vi "McPherson Control.vi"() -> ()   [LabVIEW 2020]
uses:
  Globals and TypeDefs/Type Definitions.llb/McPherson Status.ctt
  Globals and TypeDefs/Type Definitions.llb/Wavelength Unit.ctt
  Globals and TypeDefs/Type Definitions.llb/McPherson Grating Density.ctl
  Globals and TypeDefs/Error Categories.ctt
  Globals and TypeDefs/gSpectrometer.vi
  Instance          17 25Saved   McPherson Control .vi
panel:
  in  "Case Constant\n(See Context Help)":bool
  in  "Spectrometer Pos":T2
  in  "Done":bool
  in  "Tab Control":enum32{"Regular Display", "For Experts ONLY"}(tab)
  out "Speed":dbl=10.0 caption="nm/s" format="%#_3g"
  out "Lambda Chart":dbl(graph)
  in  "Grating  (g/mm)":T3=enum."1200" caption="Grating Density"
  in  "Wavelength Unit":T4=enum."nm"
  in  "Key in":bool
  out "Counter Reading":dbl=6000.0 min=0.0 max=26000.0 format="%_8f"
  out "CurrentPosition":dbl caption="nm" format="%_7f"
  out "McPherson Status":T1
  in  "Cancel":bool
  in  "Pause":bool
  in  "Scan":bool
  in  "Stop@End?":bool caption="Return to the Begin \nAFTER scan?"
  in  "Time":dbl=60.0 caption="sec" min=0.19074068422498244 format="%.2f"
  in  "End":dbl=610.0 caption="meV" format="%.3f"
  in  "Begin":dbl=600.0 caption="meV" format="%.3f"
  in  "GOTO":dbl=600.0 caption="New Position" format="%#_7f"
  in  "Slew":bool
  in  "SleepTimer Reset":bool
  out "G/U Changed?":bool
  out "Min Scan Time":dbl format="%.2f"
  in  "MiniLoop":T5(ring)
  in  "msec for actions":u32=300
  out "Time Lapse (msec)":u32(graph)
  in  "msec between z0 in scan":u32
  in  "msec between z0 in slew":u32
  in  "Wait in z0":u32=50 min=10 max=2000
  in  "PostScanSlew?":bool
  out "StepperGotoZ":i32
  out "error out":errorcluster
  out "Prior Status":T1
  out "Scan Speed":i32
  out "ScanStepperPos":T6
  # "McPherson Status"
  # "Scan"
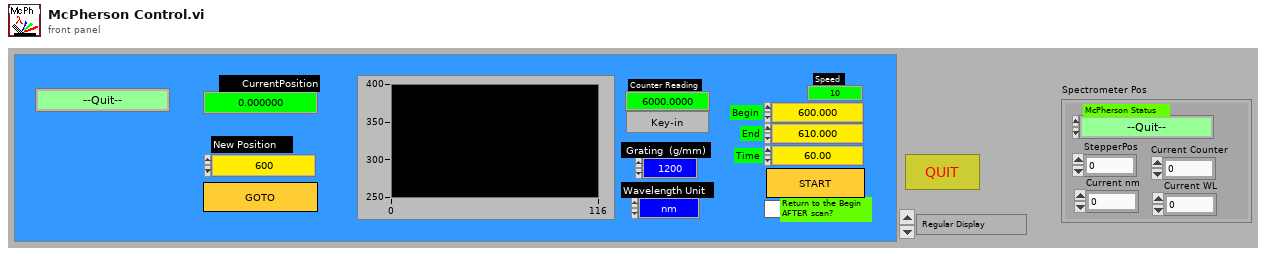
[diagram p1: front panel]
types:
  T1 = typedef "McPherson Status.ctt" = enum8{"--Quit--", "Error", "Initialization", "Standby", "Start Slew", "-Slew", "+Slew", "Slew Done", "Start Scan", "-Slew to Start", "+Slew to Start", "Scanning", "Scan Done", "Scan Pause", "Slew Pause", "Cancel", "Update Z0", "Sleep"}
  T2 = cluster{"StepperPos":i32, "Current nm":dbl, "Current Counter":dbl, "Current WL":dbl, "McPherson Status":T1}
  T3 = typedef "McPherson Grating Density.ctl" = enum8{"150", "300", "600", "1200", "1800"}
  T4 = typedef "Wavelength Unit.ctt" = enum8{"Point", "nm", "eV", "meV", "cm_1"}
  T5 = enum16{"--Exit--", "Check Parameter Changes", "Update Changes"}
  T6 = cluster{"BeginStep":i32, "EndStep":i32, "Speed Output":i16}
  T7 = typedef "Error Categories.ctt" = enum8{"General", "CCD-256x1024", "CCD-1340x400", "InGaAs PDA", "McPherson 2075", "Magnetic Field", "Temperature Control", "Other"}
  T8 = enum8{"Initialization Error", "Command Error", "Parameter Error", "Overflow Error", "Time-out Error", "Misc Error", "User cancel"}
  T9 = enum16{"Grab Globals", "Full (X, ^, Z0)", "Moving(^ and Z0)", "Position(Z0)"}
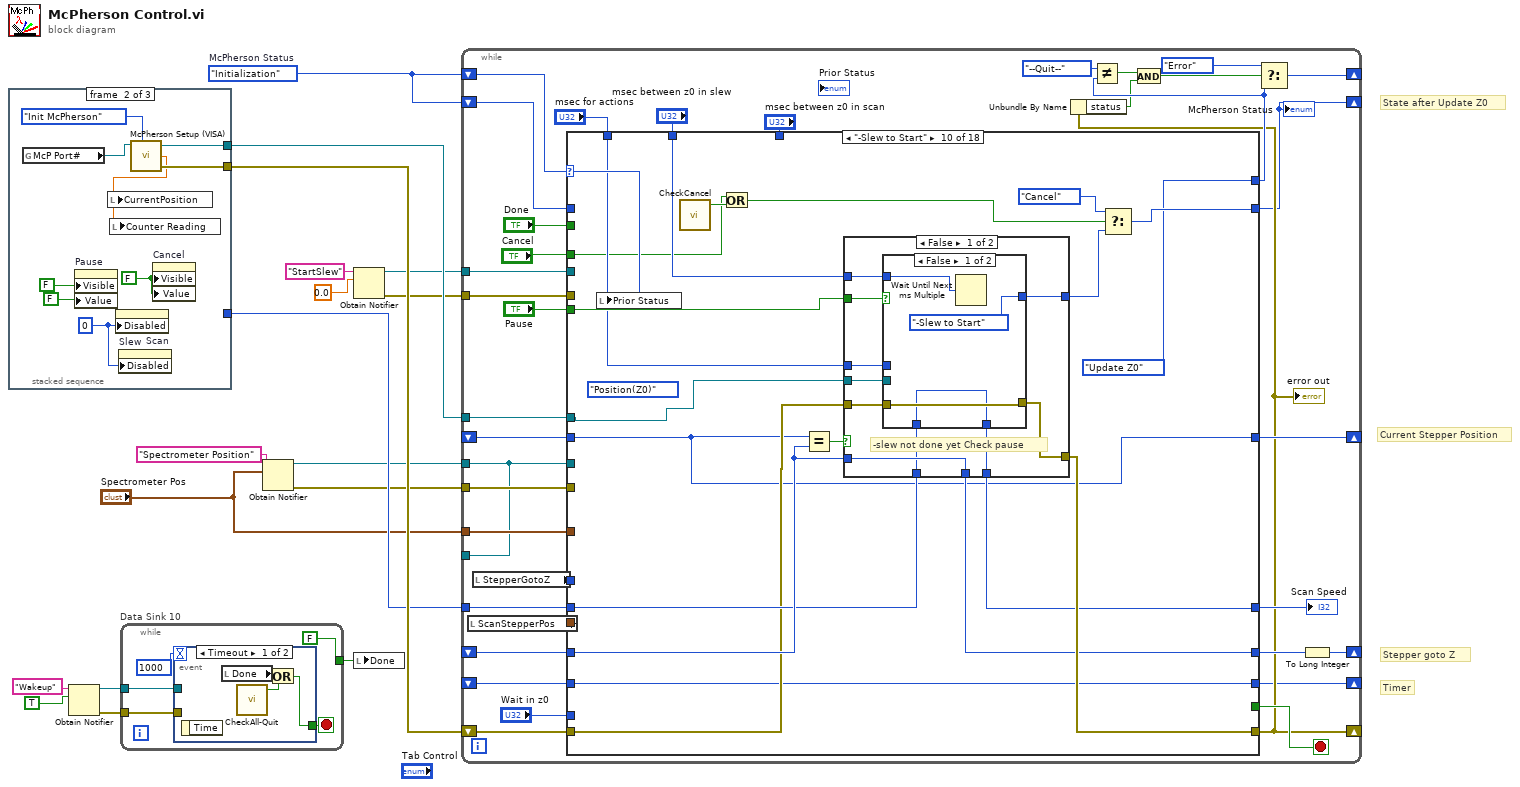
[diagram p0: block diagram]
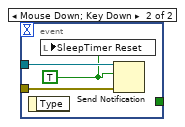
[diagram p2: hidden frame]
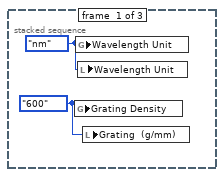
[diagram p3: hidden frame]
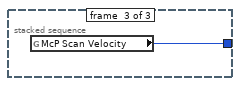
[diagram p4: hidden frame]
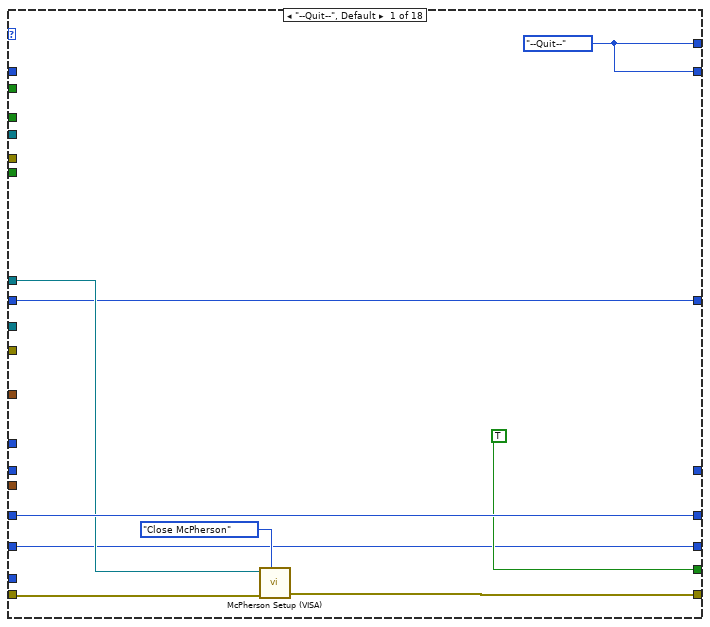
[diagram p5: hidden frame]
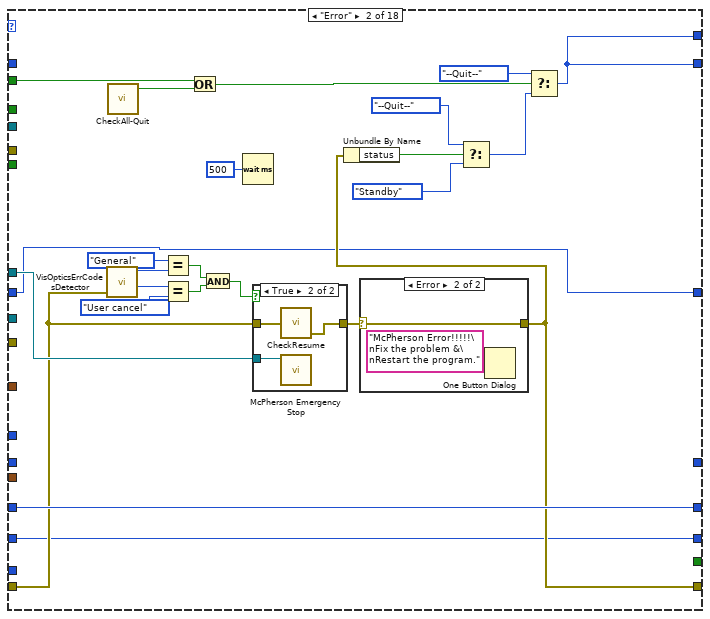
[diagram p6: hidden frame]
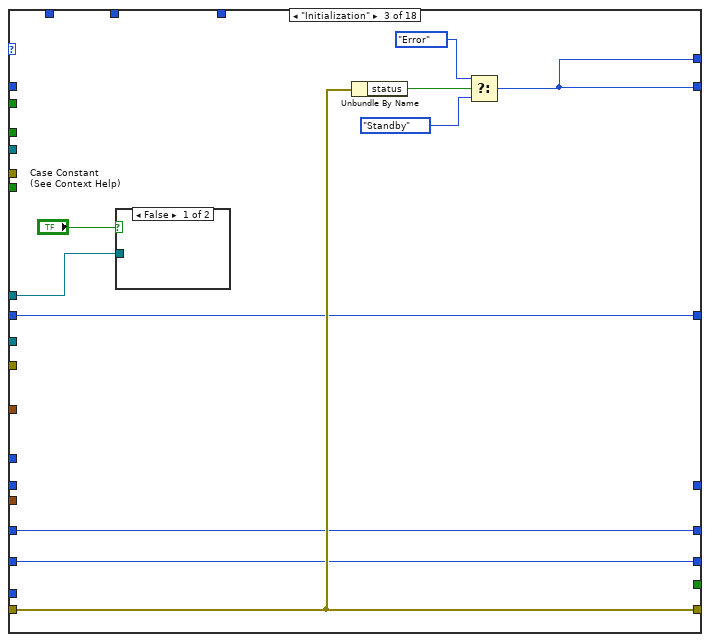
[diagram p9: hidden frame]
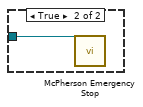
[diagram p10: hidden frame]
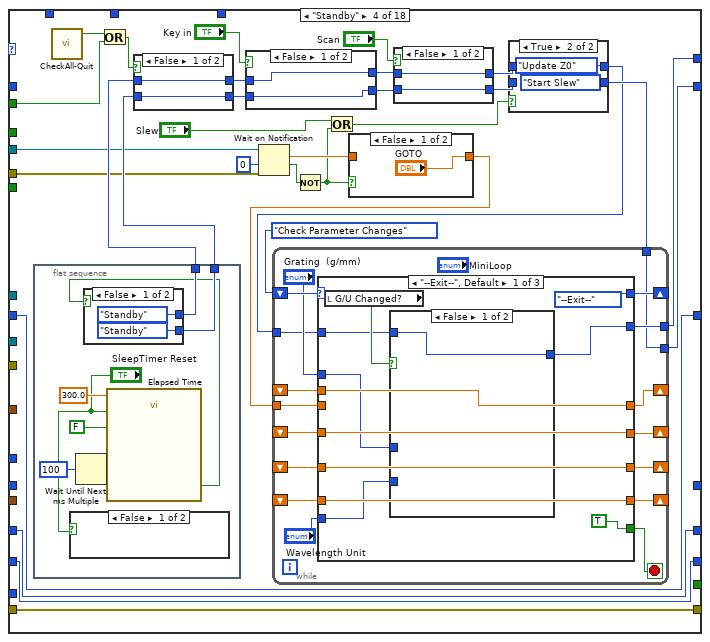
[diagram p11: hidden frame]
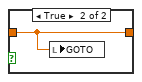
[diagram p12: hidden frame]
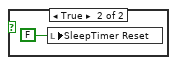
[diagram p13: hidden frame]
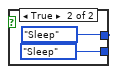
[diagram p14: hidden frame]
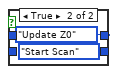
[diagram p16: hidden frame]
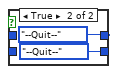
[diagram p17: hidden frame]
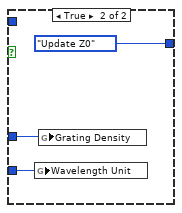
[diagram p18: hidden frame]
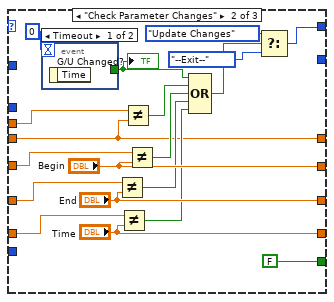
[diagram p19: hidden frame]
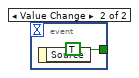
[diagram p20: hidden frame]
diagram:
  w14 = McPherson_Status.ctt."Initialization"  # McPherson Status
  # "Timer"
  # "Current Stepper Position"
  # "Stepper goto Z"
  # "State after Update Z0"
  n1 = stacked-sequence {
    tunnel: [_ w27 _] -> w17
    tunnel: [_ w26 _] -> w16
    tunnel: [_ _ w29] -> w15
    frame #0 {
      w18 = McPherson_Grating_Density."600" ("Grating Density")
      w19 = Wavelength_Unit.ctt."nm" ("Wavelength Unit")
      n2 = global write "gSpectrometer.vi" "Grating Density"(w18) -> ()
      n3 = global write "gSpectrometer.vi" "Wavelength Unit"(w19) -> ()
      n4 = local write "Wavelength Unit"(w19) -> ()
      n5 = local write "Grating  (g/mm)"(w18) -> ()
    }
    frame #1 {
      w22 = u8 0 ("Disabled")
      w21 = FALSE ("Visible")
      n6 = global read "gSpectrometer.vi" "McP Port#"() -> (w20:refnum<visa-resource-name>)
      n7 = property on="Pause" class="Bool (strict)"("Visible"=FALSE, "Value"=FALSE ("Pause")) -> ()  [unwired: 2 in, 2 out]
      n8 = property on="Scan" class="Bool"("Disabled"=w22) -> ()  [unwired: 2 in, 2 out]
      n9 = property on="Slew" class="Bool"("Disabled"=w22) -> ()  [unwired: 2 in, 2 out]
      n10 = call "McPherson Setup (VISA).vi"("VISA Resource Name"=w20, "Action"=enum8{"Init McPherson", "Close McPherson"}."Init McPherson") -> ("dup VISA Resource Name"=w27:refnum<visa-resource-name>, "Setpoint"=w25:dbl, "error out"=w26:errorcluster)  [unwired: 3 in]
      n11 = local write "CurrentPosition"(w25) -> ()
      n12 = local write "Counter Reading"(w25) -> ()
      n13 = property on="Cancel" class="Bool (strict)"("Visible"=w21, "Value"=w21) -> ()  [unwired: 2 in, 2 out]
    }
    frame #2 {
      n14 = global read "gSpectrometer.vi" "McP Scan Velocity"() -> (w29:i32)
    }
  }
  n15 = Obtain Notifier(name (unnamed)="Wakeup", notification data type=TRUE) -> (notifier out=w7:refnum<notifier>, error out=w8:errorcluster)  [unwired: 2 in, 1 out]
  n16 = while "Data Sink 10" {
    tunnel: w7 -> [w32]
    tunnel: w8 -> [w33]
    tunnel: [FALSE ("force destroy? (F)")] -> w5
    stop <- w31 stop-if-true
    n17 = event shown="[0] Timeout" {
      selector: _ -> [_ _]
      dyn-events: _ -> [_ _]
      timeout: 1000 -> [_ _]
      tunnel: w33 -> [_ w39]
      tunnel: w32 -> [_ w40]
      tunnel: [w35 _] -> w31
      event Timeout {
        n18 = event-data() -> ()  [unwired: 1 in, 1 out]
        n19 = local read "Done"() -> (w37:bool)
        n20 = call "CheckAll-Quit.vi"() -> ("All-Quit"=w36:bool)  [unwired: 3 in]
        n21 = Or(x=w37, y=w36) -> (x .or. y?=w35:bool)
      }
      event Mouse Down; Key Down {
        w38 = TRUE ("notification")
        n22 = event-data() -> ()  [unwired: 1 in, 1 out]
        n23 = local write "SleepTimer Reset"(w38) -> ()
        n24 = Send Notification(notification=w38, notifier=w40, error in (no error)=w39) -> ()  [unwired: 2 out]
      }
    }
  }
  n25 = Obtain Notifier(name (unnamed)="Spectrometer Position", notification data type="Spectrometer Pos") -> (notifier out=w12:refnum<notifier>, error out=w11:errorcluster)  [unwired: 2 in, 1 out]
  n26 = Obtain Notifier(name (unnamed)="StartSlew", notification data type=0.0) -> (notifier out=w2:refnum<notifier>, error out=w1:errorcluster)  [unwired: 2 in, 1 out]
  n27 = local write "Done"(w5) -> ()
  n28 = while {
    shift-right: [w73] -> _
    shift-left: _ -> [w76]
    tunnel: w17 -> [w68]
    shift-right: [w49] -> _
    shift-left: w16 -> [w67]
    shift-right: [w70] -> _
    shift-left: w14 -> [w71]
    shift-right: [w47] -> _
    shift-left: _ -> [w48]
    tunnel: w15 -> [w65]
    shift-right: [w43] -> _
    shift-left: w14 -> [w60]
    shift-right: [w59] -> _
    shift-left: _ -> [w58]
    tunnel: w12 -> [w44]
    tunnel: w11 -> [w46]
    tunnel: "Spectrometer Pos" -> [w45]
    tunnel: [w44] -> _
    tunnel: w2 -> [w42]
    tunnel: w1 -> [w41]
    stop <- w77 stop-if-true
    n29 = local read "ScanStepperPos"() -> (w57:T6)
    n30 = local read "StepperGotoZ"() -> (w56:i32)
    n31 = case shown="\"-Slew to Start\"" w71 {
      selector: w71 -> [_ _ _ _ _ w328 w380 _ _ w495 w548 _ _ _ _ _ _ _]
      tunnel: [TRUE _ _ _ _ _ _ _ _ _ _ _ _ _ _ _ _ _] -> w77
      tunnel: [w86 w107 w122 w159 w273 w326 w373 w414 w441 w493 w539 w602 w644 w668 w693 w723 w742 w779] -> w74
      tunnel: w76 -> [w86 w107 w122 w159 _ w327 w373 w414 _ w494 w539 w602 w644 w668 w693 w723 w742 w779]
      tunnel: w68 -> [w84 w101 w124 _ w263 w316 w369 _ w430 w485 w535 w587 _ w670 w699 w724 w745 _]
      tunnel: w67 -> [w82 w95 w123 w155 w262 w317 w370 w412 w429 w484 w536 w588 w642 w671 w700 w725 w744 w774]
      tunnel: [w81 w93 w123 w155 w274 w330 w377 w412 w444 w497 w545 w606 w642 w669 w698 w718 w743 w774] -> w49
      tunnel: "Pause" -> [_ _ _ _ _ w329 w381 _ _ w496 w549 w603 _ w667 w697 _ _ _]
      tunnel: [w78 w88 w119 w140 w259 McPherson_Status.ctt."Update Z0" ("McPherson Status") w366 McPherson_Status.ctt."Update Z0" ("McPherson Status") McPherson_Status.ctt."Update Z0" ("McPherson Status") McPherson_Status.ctt."Update Z0" ("McPherson Status") McPherson_Status.ctt."Update Z0" ("McPherson Status") McPherson_Status.ctt."Update Z0" ("McPherson Status") McPherson_Status.ctt."Update Z0" ("McPherson Status") w666 w696 McPherson_Status.ctt."Update Z0" ("McPherson Status") w726 McPherson_Status.ctt."Standby" ("McPherson Status")] -> w55
      tunnel: "Cancel" -> [_ _ _ _ _ w312 w364 _ w424 w479 w530 w582 w637 w657 w686 _ _ _]
      tunnel: w56 -> [_ _ _ _ w268 _ _ _ _ _ _ _ _ _ _ _ _ _]
      tunnel: w57 -> [_ _ _ _ w270 _ _ _ w439 _ w543 w595 _ w664 _ _ _ _]
      tunnel: "Done" -> [_ w91 _ w157 _ _ _ _ _ _ _ _ _ _ _ _ _ _]
      tunnel: [_ _ _ _ w271 w322 w375 _ w437 w488 w541 w591 _ w663 w691 _ w730 _] -> w66
      tunnel: w65 -> [_ _ _ _ w271 w321 w374 _ w436 w489 w540 _ _ _ w692 _ _ _]
      tunnel: "Wait in z0" -> [_ _ _ _ _ _ _ _ _ _ _ _ _ _ _ _ w741 _]
      tunnel: "msec between z0 in slew" -> [_ _ _ _ _ w320 w372 _ _ w487 w538 _ _ _ _ _ _ _]
      tunnel: "msec between z0 in scan" -> [_ _ _ _ _ _ _ _ _ _ _ w590 _ _ _ _ _ _]
      tunnel: "msec for actions" -> [_ _ _ _ w265 w319 w371 _ w435 w486 w537 w589 _ w662 w690 w721 _ _]
      tunnel: [w78 w88 w119 w141 w260 w318 w368 McPherson_Status.ctt."Standby" ("McPherson Status") w427 w482 w533 w585 w640 w660 w689 McPherson_Status.ctt."Slew Done" ("McPherson Status") w726 McPherson_Status.ctt."Standby" ("McPherson Status")] -> w43
      tunnel: w60 -> [_ _ _ _ _ _ _ _ _ _ _ _ _ _ _ _ w735 _]
      tunnel: [w80 w89 w120 w145 w261 w314 w367 w411 w428 w483 w534 w586 w641 w659 w688 w717 w731 w777] -> w59
      tunnel: w58 -> [w80 w89 w120 w145 w261 w314 w367 w411 w428 w483 w534 w586 w641 w659 w688 w717 _ w777]
      tunnel: w48 -> [w79 w87 w118 w154 w258 w310 w362 w409 w422 w477 w528 w580 w635 w655 w684 w715 w733 w775]
      tunnel: [w79 w87 w118 w154 w258 w310 w362 w409 w422 w477 w528 w580 w635 w655 w684 w715 w732 w775] -> w47
      tunnel: w44 -> [_ _ _ _ _ _ _ _ _ _ _ _ _ _ _ _ w729 _]
      tunnel: w46 -> [_ _ _ _ _ _ _ _ _ _ _ _ _ _ _ _ w728 _]
      tunnel: w45 -> [_ _ _ _ _ _ _ _ _ _ _ _ _ _ _ _ w727 _]
      tunnel: w42 -> [_ _ _ w130 _ _ _ _ _ _ _ _ _ _ _ _ _ _]
      tunnel: w41 -> [_ _ _ w129 _ _ _ _ _ _ _ _ _ _ _ _ _ _]
      frame "--Quit--", Default {
        w78 = McPherson_Status.ctt."--Quit--"
        n32 = call "McPherson Setup (VISA).vi"("VISA Resource Name"=w84, "error in"=w82, "Action"=enum8{"Init McPherson", "Close McPherson"}."Close McPherson") -> ("error out"=w81:errorcluster)  [unwired: 2 in, 2 out]
      }
      frame "Error" {
        n33 = call "VisOpticsErrCodesDetector.vi"("error in"=w95) -> ("NHMFL Visible Optics Error Category"=w100:T7, "NHMFL Visible Optics Error Type"=w103:T8)  [unwired: 2 in, 2 out]
        n34 = call "CheckAll-Quit.vi"() -> ("All-Quit"=w92:bool)  [unwired: 3 in]
        n35 = Equal?(x=Error_Categories.ctt."General", y=w100) -> (x = y?=w98:bool)
        n36 = Equal?(x=w103, y=T8."User cancel") -> (x = y?=w97:bool)
        n37 = Or(x=w91, y=w92) -> (x .or. y?=w90:bool)
        n38 = And(x=w98, y=w97) -> (x .and. y?=w96:bool)
        n39 = Wait (ms)(milliseconds to wait=u32 500) -> ()  [unwired: 1 out]
        n40 = case shown="True" w96 {
          tunnel: w101 -> [_ w117]
          tunnel: w95 -> [w114 w116]
          tunnel: [w114 w115] -> w94
          frame False {
          }
          frame True {
            n41 = call "CheckResume.vi"("error in"=w116) -> ("error out"=w115:errorcluster)  [unwired: 1 in, 1 out]
            n42 = call "McPherson Emergency Stop.vi"("VISA Resource Name"=w117) -> ()  [unwired: 4 in, 2 out]
          }
        }
        n43 = case shown="Error" w94 {
          selector: w94 -> [w111 w113]
          tunnel: [w111 w113] -> w93
          frame No Error {
          }
          frame Error {
            n44 = One Button Dialog(message="McPherson Error!!!!!\nFix the problem &\nRestart the program.") -> ()  [unwired: 1 in, 1 out]
          }
        }
        n45 = Unbundle By Name(w93) -> ("status"=w110:bool)
        n46 = Select(t=McPherson_Status.ctt."--Quit--", s=w110, f=McPherson_Status.ctt."Standby" ("McPherson Status")) -> (s? t:f=w106:T1)
        n47 = Select(t=McPherson_Status.ctt."--Quit--", s=w90, f=w106) -> (s? t:f=w88:T1)
      }
      frame "Initialization" {
        n48 = case shown="False" "Case Constant\n(See Context Help)" {
          tunnel: w124 -> [_ w128]
          frame False {
          }
          frame True {
            n49 = call "McPherson Emergency Stop.vi"("VISA Resource Name"=w128) -> ()  [unwired: 4 in, 2 out]
          }
        }
        n50 = Unbundle By Name(w123) -> ("status"=w127:bool)
        n51 = Select(t=McPherson_Status.ctt."Error", s=w127, f=McPherson_Status.ctt."Standby" ("McPherson Status")) -> (s? t:f=w119:T1)
      }
      frame "Standby" {
        n52 = flat-sequence {
          tunnel: [w165] -> w144
          tunnel: [w164] -> w143
          frame #0 {
            n53 = case shown="False" "SleepTimer Reset" {
              frame False {
              }
              frame True {
                n54 = local write "SleepTimer Reset"(FALSE ("SleepTimer Reset")) -> ()
              }
            }
            n55 = Wait Until Next ms Multiple(millisecond multiple=u32 100) -> ()  [unwired: 1 out]
            n56 = call "Elapsed Time"("Time Target (s)"=300.0, "Reset"="SleepTimer Reset", "Auto Reset"=FALSE) -> ("Time has Elapsed"=w162:bool)  [unwired: 9 in, 7 out]
            n57 = case shown="False" w162 {
              tunnel: [McPherson_Status.ctt."Standby" ("McPherson Status") McPherson_Status.ctt."Sleep" ("McPherson Status")] -> w165
              tunnel: [McPherson_Status.ctt."Standby" ("McPherson Status") McPherson_Status.ctt."Sleep" ("McPherson Status")] -> w164
              frame False {
              }
              frame True {
              }
            }
          }
        }
        n58 = call "CheckAll-Quit.vi"() -> ("All-Quit"=w131:bool)  [unwired: 3 in]
        n59 = Or(x=w131, y=w157) -> (x .or. y?=w153:bool)
        n60 = case shown="False" w153 {
          tunnel: [w183 McPherson_Status.ctt."--Quit--" ("McPherson Status")] -> w152
          tunnel: [w182 McPherson_Status.ctt."--Quit--" ("McPherson Status")] -> w151
          tunnel: w144 -> [w183 _]
          tunnel: w143 -> [w182 _]
          frame False {
          }
          frame True {
          }
        }
        n61 = case shown="False" "Key in" {
          tunnel: w152 -> [w254 _]
          tunnel: [w254 McPherson_Status.ctt."Update Z0" ("McPherson Status")] -> w150
          tunnel: [w253 McPherson_Status.ctt."Standby" ("McPherson Status")] -> w149
          tunnel: w151 -> [w253 _]
          frame False {
          }
          frame True {
            n62 = call "KeyInCounterPosition.vi"() -> ()  [unwired: 1 in, 2 out]
          }
        }
        n63 = Wait on Notification(notifier=w130, timeout in ms (-1)=0, error in (no error)=w129) -> (notification=w136:dbl, timed out?=w137:bool)  [unwired: 1 in, 2 out]
        n64 = Not(x=w137) -> (.not. x?=w134:bool)
        n65 = Or(x="Slew", y=w134) -> (x .or. y?=w132:bool)
        n66 = case shown="False" w134 {
          tunnel: w136 -> [_ w161]
          tunnel: ["GOTO" w161] -> w135
          frame False {
          }
          frame True {
            n67 = local write "GOTO"(w161) -> ()
          }
        }
        n68 = case shown="False" "Scan" {
          tunnel: [w179 McPherson_Status.ctt."Update Z0" ("McPherson Status")] -> w147
          tunnel: [w178 McPherson_Status.ctt."Start Scan" ("McPherson Status")] -> w146
          tunnel: w150 -> [w179 _]
          tunnel: w149 -> [w178 _]
          frame False {
          }
          frame True {
          }
        }
        n69 = case shown="True" w132 {
          tunnel: [w175 McPherson_Status.ctt."Update Z0" ("McPherson Status")] -> w139
          tunnel: [w174 McPherson_Status.ctt."Start Slew" ("McPherson Status")] -> w142
          tunnel: w147 -> [w175 _]
          tunnel: w146 -> [w174 _]
          frame False {
          }
          frame True {
          }
        }
        n70 = while {
          shift-right: [w195] -> _
          shift-left: _ -> [w194]
          shift-right: [w197] -> _
          shift-left: _ -> [w196]
          shift-right: [w199] -> _
          shift-left: _ -> [w198]
          shift-right: [w200] -> _
          shift-left: _ -> [w201]
          shift-right: [w193] -> _
          shift-left: T5."Check Parameter Changes" ("MiniLoop") -> [w202]
          tunnel: [w189] -> w140
          tunnel: [w188] -> w141
          tunnel: w142 -> [w188]
          tunnel: w139 -> [w187]
          tunnel: w135 -> [w186]
          stop <- w190 stop-if-true
          n71 = case shown="\"--Exit--\", Default" w202 {
            tunnel: w201 -> [w210 w235 w242]
            tunnel: [w210 "Time" w242] -> w200
            tunnel: [w211 "End" w243] -> w199
            tunnel: w198 -> [w211 w232 w246]
            tunnel: [w212 "Begin" w244] -> w197
            tunnel: w196 -> [w212 w230 w247]
            tunnel: [w213 w218 w245] -> w195
            tunnel: w194 -> [w213 w229 w248]
            tunnel: [T5."--Exit--" ("MiniLoop") w221 T5."--Exit--" ("MiniLoop")] -> w193
            tunnel: "Grating  (g/mm)" -> [w205 _ w250]
            tunnel: "Wavelength Unit" -> [w204 _ w249]
            tunnel: [TRUE ("G/U Changed?") FALSE ("G/U Changed?") FALSE ("G/U Changed?")] -> w190
            tunnel: [w206 _ _] -> w189
            tunnel: w187 -> [w203 _ _]
            tunnel: w186 -> [_ w218 _]
            frame "--Exit--", Default {
              n72 = local read "G/U Changed?"() -> (w207:bool)
              n73 = case shown="False" w207 {
                tunnel: [w214 McPherson_Status.ctt."Update Z0" ("McPherson Status")] -> w206
                tunnel: w205 -> [_ w217]
                tunnel: w204 -> [_ w216]
                tunnel: w203 -> [w214 _]
                frame False {
                }
                frame True {
                  n74 = global write "gSpectrometer.vi" "Wavelength Unit"(w216) -> ()
                  n75 = global write "gSpectrometer.vi" "Grating Density"(w217) -> ()
                }
              }
            }
            frame "Check Parameter Changes" {
              n76 = event shown="[0] Timeout" {
                selector: _ -> [_ _]
                dyn-events: _ -> [_ _]
                timeout: 0 -> [_ _]
                tunnel: [_ TRUE ("Done")] -> w219
                event Timeout {
                  n77 = event-data() -> ()  [unwired: 1 in, 1 out]
                }
                event Value Change {
                  n78 = event-data() -> ()  [unwired: 1 in, 1 out]
                }
              }
              "G/U Changed?" <- w219
              n79 = Not Equal?(x=w232, y="End") -> (x != y?=w226:bool)
              n80 = Not Equal?(x=w235, y="Time") -> (x != y?=w225:bool)
              n81 = Not Equal?(x=w229, y=w218) -> (x != y?=w228:bool)
              n82 = Not Equal?(x=w230, y="Begin") -> (x != y?=w227:bool)
              n83 = Compound Arithmetic op=OR(w219, w228, w227, w226, w225) -> (w224:bool)
              n84 = Select(t=T5."Update Changes", s=w224, f=T5."--Exit--" ("MiniLoop")) -> (s? t:f=w221:T5)
            }
            frame "Update Changes" {
              n85 = call "McPherson Setup for new pi.vi"("Old GOTO"=w248, "Old Begin"=w247, "Old End"=w246, "Duration"=w242, "New Wavelength Unit"=w249, "Grating Density (g/mm)"=w250) -> ("Min Scan Time"=w251:dbl, "StepperOutput"=→"ScanStepperPos":T6, "New GOTO"=w245:dbl, "New Begin"=w244:dbl, "New End"=w243:dbl, "StepperGotoZ"=→"StepperGotoZ":i32)  [unwired: 7 in, 1 out]
              "Min Scan Time" <- w251
              n86 = local write "GOTO"(w245) -> ()
              n87 = local write "Begin"(w244) -> ()
              n88 = local write "End"(w243) -> ()
              n89 = property on="Time" class="DigNum (strict)"("Data Range:Minimum"=w251, "Out Of Range Action:Minimum"=u8 1) -> ()  [unwired: 2 in, 2 out]
            }
          }
        }
      }
      frame "Start Slew" {
        n90 = Unbundle By Name(w270) -> ("BeginStep"=w269:i32)
        n91 = case shown="False" "PostScanSlew?" {
          tunnel: w269 -> [_ w279]
          tunnel: w268 -> [w276 _]
          tunnel: [w276 w279] -> w267
          tunnel: [w275 w277] -> w264
          frame False {
            n92 = local read "GOTO"() -> (w275:dbl)
          }
          frame True {
            n93 = local read "Begin"() -> (w277:dbl)
            n94 = local write "PostScanSlew?"(FALSE ("PostScanSlew?")) -> ()
          }
        }
        n95 = Equal?(x=w261, y=w267) -> (x = y?=w272:bool)
        n96 = case shown="False" w272 {
          tunnel: w261 -> [w304 w308]
          tunnel: w267 -> [w300 _]
          tunnel: w263 -> [w303 _]
          tunnel: w262 -> [w291 w309]
          tunnel: [w292 w309] -> w274
          tunnel: [w296 w307] -> w260
          tunnel: [w295 w308] -> w273
          tunnel: w265 -> [w290 _]
          tunnel: w264 -> [w284 _]
          tunnel: [McPherson_Status.ctt."Update Z0" ("McPherson Status") w307] -> w259
          frame False {
            w289 = u8 2 ("Disabled")
            n97 = local read "CurrentPosition"() -> (w283:dbl)
            n98 = Subtract(x=w300, y=5000) -> (x-y=w299:i32)
            n99 = property on="Scan" class="Bool"("Disabled"=w289) -> ()  [unwired: 2 in, 2 out]
            n100 = property on="Slew" class="Bool"("Disabled"=w289) -> ()  [unwired: 2 in, 2 out]
            n101 = Less?(x=w304, y=w300) -> (x < y?=w302:bool)
            n102 = Max & Min(x=w283, y=w284) -> (max(x,y)=w282:dbl, min(x,y)=w281:dbl)
            n103 = Select(t=w300, s=w302, f=w299) -> (s? t:f=w295:i32)
            n104 = Select(t=McPherson_Status.ctt."+Slew" ("McPherson Status"), s=w302, f=McPherson_Status.ctt."-Slew" ("McPherson Status")) -> (s? t:f=w296:T1)
            n105 = property on="Pause" class="Bool (strict)"("Visible"=TRUE, "Value"=FALSE ("Pause")) -> ()  [unwired: 2 in, 2 out]
            n106 = property on="Lambda Chart" class="WFChart (strict)"("Y Scale.Range:Maximum"=w282, "Y Scale.Range:Minimum"=w281) -> ()  [unwired: 2 in, 2 out]
            n107 = call "McPherson Set X V.vi"("VISA Resource Name"=w303, "milliseconds to wait"=w290, "SetValue In"=w295, "error In"=w291, "Action"=enum16{"Stop", "MoveTo", "SpeedAt"}."MoveTo") -> ("error out"=w293:errorcluster)  [unwired: 2 out]
            n108 = flat-sequence {
              tunnel: [w306] -> w292
              tunnel: w293 -> [w306]
              frame #0 {
                n109 = Wait (ms)(milliseconds to wait=u32 100) -> ()  [unwired: 1 out]
              }
            }
            n110 = property on="Cancel" class="Bool (strict)"("Visible"=TRUE, "Value"=FALSE ("Cancel")) -> ()  [unwired: 2 in, 2 out]
          }
          frame True {
            w307 = McPherson_Status.ctt."Slew Done" ("McPherson Status")
          }
        }
        n111 = local write "SleepTimer Reset"(TRUE ("SleepTimer Reset")) -> ()
      }
      frame "-Slew" {
        n112 = local write "Prior Status"(w328) -> ()
        n113 = call "CheckCancel.vi"() -> ("Cancelled"=w313:bool)  [unwired: 2 in, 1 out]
        n114 = Or(x=w312, y=w313) -> (x .or. y?=w311:bool)
        n115 = Equal?(x=w314, y=w327) -> (x = y?=w325:bool)
        n116 = case shown="True" w325 {
          tunnel: w316 -> [w336 w360]
          tunnel: w317 -> [w337 w361]
          tunnel: [w335 w356] -> w330
          tunnel: w329 -> [w340 _]
          tunnel: w327 -> [w338 w359]
          tunnel: [w338 w357] -> w326
          tunnel: [w339 McPherson_Status.ctt."+Slew" ("McPherson Status")] -> w323
          tunnel: [w334 w354] -> w322
          tunnel: w321 -> [w333 w354]
          tunnel: w320 -> [w332 _]
          tunnel: w319 -> [w331 w352]
          frame False {
            # "-slew not done yet Check pause"
            n117 = case shown="True" w340 {
              tunnel: [McPherson_Status.ctt."-Slew" ("McPherson Status") McPherson_Status.ctt."Slew Pause" ("McPherson Status")] -> w339
              tunnel: w337 -> [w343 w350]
              tunnel: w336 -> [_ w348]
              tunnel: [w343 w347] -> w335
              tunnel: [w342 0 ("McP Scan Velocity")] -> w334
              tunnel: w333 -> [w342 _]
              tunnel: w332 -> [w341 _]
              tunnel: w331 -> [_ w345]
              frame False {
                n118 = Wait Until Next ms Multiple(millisecond multiple=w341) -> ()  [unwired: 1 out]
              }
              frame True {
                n119 = call "McPherson Set X V.vi"("VISA Resource Name"=w348, "milliseconds to wait"=w345, "error In"=w350, "Action"=enum16{"Stop", "MoveTo", "SpeedAt"}."Stop") -> ("error out"=w347:errorcluster)  [unwired: 1 in, 2 out]
              }
            }
          }
          frame True {
            # "-slew done \nadd 5000 and +slew\nto reset backlash"
            n120 = Add(x=5000, y=w359) -> (x+y=w357:i32)
            n121 = call "McPherson Set X V.vi"("VISA Resource Name"=w360, "milliseconds to wait"=w352, "SetValue In"=w357, "error In"=w361, "Action"=enum16{"Stop", "MoveTo", "SpeedAt"}."MoveTo") -> ("error out"=w356:errorcluster)  [unwired: 2 out]
          }
        }
        n122 = Select(t=McPherson_Status.ctt."Cancel" ("McPherson Status"), s=w311, f=w323) -> (s? t:f=w318:T1)
      }
      frame "+Slew" {
        n123 = local write "Prior Status"(w380) -> ()
        n124 = call "CheckCancel.vi"() -> ("Cancelled"=w365:bool)  [unwired: 2 in, 1 out]
        n125 = Or(x=w364, y=w365) -> (x .or. y?=w363:bool)
        n126 = Equal?(x=w367, y=w373) -> (x = y?=w379:bool)
        n127 = case shown="True" w379 {
          tunnel: w369 -> [w387 _]
          tunnel: w381 -> [w391 _]
          tunnel: [w390 w403] -> w376
          tunnel: w370 -> [w389 w405]
          tunnel: [w388 w405] -> w377
          tunnel: [w386 0] -> w375
          tunnel: w374 -> [w385 _]
          tunnel: w372 -> [w384 _]
          tunnel: w371 -> [w383 _]
          tunnel: [McPherson_Status.ctt."Update Z0" ("McPherson Status") w403] -> w366
          frame False {
            # "+slew not done yet\nCheck pause"
            n128 = case shown="True" w391 {
              tunnel: [McPherson_Status.ctt."+Slew" ("McPherson Status") McPherson_Status.ctt."Slew Pause" ("McPherson Status")] -> w390
              tunnel: w389 -> [w394 w401]
              tunnel: [w394 w400] -> w388
              tunnel: w387 -> [_ w399]
              tunnel: [w393 i16 0 ("Scan Speed")] -> w386
              tunnel: w385 -> [w393 _]
              tunnel: w384 -> [w392 _]
              tunnel: w383 -> [_ w396]
              frame False {
                n129 = Wait Until Next ms Multiple(millisecond multiple=w392) -> ()  [unwired: 1 out]
              }
              frame True {
                n130 = call "McPherson Set X V.vi"("VISA Resource Name"=w399, "milliseconds to wait"=w396, "error In"=w401, "Action"=enum16{"Stop", "MoveTo", "SpeedAt"}."Stop") -> ("error out"=w400:errorcluster)  [unwired: 1 in, 2 out]
              }
            }
          }
          frame True {
            w403 = McPherson_Status.ctt."Slew Done" ("McPherson Status")
            # "+slew done"
          }
        }
        n131 = Select(t=McPherson_Status.ctt."Cancel" ("McPherson Status"), s=w363, f=w376) -> (s? t:f=w368:T1)
      }
      frame "Slew Done" {
        w413 = u8 0 ("Disabled")
        w408 = FALSE ("Visible")
        w407 = FALSE ("Visible")
        n132 = flat-sequence {
          frame #0 {
            n133 = Wait (ms)(milliseconds to wait=u32 100) -> ()  [unwired: 1 out]
          }
          frame #1 {
            w418 = u16 0 items=["Moving", "Calibration", "Key in", "Initialization"] ("Set Method")
            n134 = global read "gSpectrometer.vi" "CurrentStepperPosition"() -> (w416:i32)
            n135 = global read "gSpectrometer.vi" "Current Counter Position"() -> (w417:dbl)
            n136 = call "Load_McP_CounterPos.dat.VI"() -> ("Last Calibration Date"=w419:string)  [unwired: 1 in, 2 out]
            n137 = call "Save McP CounterPos.dat.VI"("Last Calibration Date"=w419, "Set Method"=w418, "McP Stepper Position"=w416, "McP Counter Position"=w417) -> ()  [unwired: 2 in, 1 out]
          }
        }
        n138 = property on="Scan" class="Bool"("Disabled"=w413) -> ()  [unwired: 2 in, 2 out]
        n139 = property on="Slew" class="Bool"("Disabled"=w413) -> ()  [unwired: 2 in, 2 out]
        n140 = property on="Pause" class="Bool (strict)"("Visible"=w407, "Value"=w407) -> ()  [unwired: 2 in, 2 out]
        n141 = property on="Cancel" class="Bool (strict)"("Visible"=w408, "Value"=w408) -> ()  [unwired: 2 in, 2 out]
      }
      frame "Start Scan" {
        w434 = u8 2 ("Disabled")
        # "Setup stepper"
        n142 = call "CheckCancel.vi"() -> ("Cancelled"=w425:bool)  [unwired: 2 in, 1 out]
        n143 = Unbundle By Name(w439) -> ("BeginStep"=w438:i32, "Speed Output"=w440:i16)
        n144 = Or(x=w424, y=w425) -> (x .or. y?=w423:bool)
        n145 = local write "SleepTimer Reset"(TRUE ("SleepTimer Reset")) -> ()
        n146 = property on="Scan" class="Bool"("Disabled"=w434) -> ()  [unwired: 2 in, 2 out]
        n147 = Equal?(x=w428, y=w438) -> (x = y?=w445:bool)
        n148 = property on="Slew" class="Bool"("Disabled"=w434) -> ()  [unwired: 2 in, 2 out]
        n149 = case shown="False" w445 {
          tunnel: w428 -> [w464 _]
          tunnel: w430 -> [w463 w473]
          tunnel: w429 -> [w462 w475]
          tunnel: [w460 w474] -> w444
          tunnel: [w455 McPherson_Status.ctt."Scanning" ("McPherson Status")] -> w443
          tunnel: [w454 w472] -> w441
          tunnel: w440 -> [_ w471]
          tunnel: w438 -> [w453 w472]
          tunnel: [w452 w471] -> w437
          tunnel: w436 -> [w452 _]
          tunnel: w435 -> [w450 w469]
          frame False {
            n150 = local read "CurrentPosition"() -> (w447:dbl)
            n151 = local read "Begin"() -> (w446:dbl)
            n152 = Subtract(x=w453, y=5000) -> (x-y=w458:i32)
            n153 = Less?(x=w464, y=w453) -> (x < y?=w461:bool)
            n154 = Max & Min(x=w447, y=w446) -> (max(x,y)=w449:dbl, min(x,y)=w448:dbl)
            n155 = Select(t=w453, s=w461, f=w458) -> (s? t:f=w454:i32)
            n156 = Select(t=McPherson_Status.ctt."+Slew to Start" ("McPherson Status"), s=w461, f=McPherson_Status.ctt."-Slew to Start" ("McPherson Status")) -> (s? t:f=w455:T1)
            n157 = property on="Lambda Chart" class="WFChart (strict)"("Y Scale.Range:Maximum"=w449, "Y Scale.Range:Minimum"=w448) -> ()  [unwired: 2 in, 2 out]
            n158 = call "McPherson Set X V.vi"("VISA Resource Name"=w463, "milliseconds to wait"=w450, "SetValue In"=w454, "error In"=w462, "Action"=enum16{"Stop", "MoveTo", "SpeedAt"}."MoveTo") -> ("error out"=w460:errorcluster)  [unwired: 2 out]
          }
          frame True {
            n159 = local read "Begin"() -> (w466:dbl)
            n160 = local read "End"() -> (w465:dbl)
            n161 = Max & Min(x=w466, y=w465) -> (max(x,y)=w468:dbl, min(x,y)=w467:dbl)
            n162 = call "McPherson Set X V.vi"("VISA Resource Name"=w473, "milliseconds to wait"=w469, "SetValue In"=w471, "error In"=w475, "Action"=enum16{"Stop", "MoveTo", "SpeedAt"}."SpeedAt") -> ("error out"=w474:errorcluster)  [unwired: 2 out]
            n163 = property on="Lambda Chart" class="WFChart (strict)"("Y Scale.Range:Maximum"=w468, "Y Scale.Range:Minimum"=w467) -> ()  [unwired: 2 in, 2 out]
          }
        }
        n164 = property on="Pause" class="Bool (strict)"("Visible"=TRUE, "Value"=FALSE ("Pause")) -> ()  [unwired: 2 in, 2 out]
        n165 = property on="Cancel" class="Bool (strict)"("Visible"=TRUE, "Value"=FALSE ("Cancel")) -> ()  [unwired: 2 in, 2 out]
        n166 = Select(t=McPherson_Status.ctt."Cancel", s=w423, f=w443) -> (s? t:f=w427:T1)
      }
      frame "-Slew to Start" {
        (unwired) T9."Position(Z0)" ("Status")
        n167 = local write "Prior Status"(w495) -> ()
        n168 = call "CheckCancel.vi"() -> ("Cancelled"=w480:bool)  [unwired: 2 in, 1 out]
        n169 = Or(x=w479, y=w480) -> (x .or. y?=w478:bool)
        n170 = Equal?(x=w483, y=w494) -> (x = y?=w492:bool)
        n171 = case shown="False" w492 {
          tunnel: w485 -> [w503 w526]
          tunnel: w484 -> [w504 w527]
          tunnel: [w502 w522] -> w497
          tunnel: w496 -> [w507 _]
          tunnel: w494 -> [w505 w525]
          tunnel: [w505 w523] -> w493
          tunnel: [w506 McPherson_Status.ctt."+Slew to Start" ("McPherson Status")] -> w490
          tunnel: w489 -> [w501 w520]
          tunnel: [w500 w520] -> w488
          tunnel: w487 -> [w499 _]
          tunnel: w486 -> [w498 w518]
          frame False {
            # "-slew not done yet Check pause"
            n172 = case shown="False" w507 {
              tunnel: [McPherson_Status.ctt."-Slew to Start" ("McPherson Status") McPherson_Status.ctt."Slew Pause" ("McPherson Status")] -> w506
              tunnel: w504 -> [w510 w516]
              tunnel: w503 -> [_ w515]
              tunnel: [w510 w514] -> w502
              tunnel: w501 -> [w509 _]
              tunnel: [w509 _] -> w500
              tunnel: w499 -> [w508 _]
              tunnel: w498 -> [_ w512]
              frame False {
                n173 = Wait Until Next ms Multiple(millisecond multiple=w508) -> ()  [unwired: 1 out]
              }
              frame True {
                n174 = call "McPherson Set X V.vi"("VISA Resource Name"=w515, "milliseconds to wait"=w512, "error In"=w516, "Action"=enum16{"Stop", "MoveTo", "SpeedAt"}."Stop") -> ("error out"=w514:errorcluster)  [unwired: 1 in, 2 out]
              }
            }
          }
          frame True {
            # "-slew done \nadd 5000 and +slew\nto reset backlash"
            n175 = Add(x=5000, y=w525) -> (x+y=w523:i32)
            n176 = call "McPherson Set X V.vi"("VISA Resource Name"=w526, "milliseconds to wait"=w518, "SetValue In"=w523, "error In"=w527, "Action"=enum16{"Stop", "MoveTo", "SpeedAt"}."MoveTo") -> ("error out"=w522:errorcluster)  [unwired: 2 out]
          }
        }
        n177 = Select(t=McPherson_Status.ctt."Cancel" ("McPherson Status"), s=w478, f=w490) -> (s? t:f=w482:T1)
      }
      frame "+Slew to Start" {
        n178 = local write "Prior Status"(w548) -> ()
        n179 = Unbundle By Name(w543) -> ("Speed Output"=w542:i16)
        n180 = call "CheckCancel.vi"() -> ("Cancelled"=w531:bool)  [unwired: 2 in, 1 out]
        n181 = Equal?(x=w534, y=w539) -> (x = y?=w547:bool)
        n182 = Or(x=w530, y=w531) -> (x .or. y?=w529:bool)
        n183 = case shown="True" w547 {
          tunnel: w535 -> [w554 w576]
          tunnel: w549 -> [w558 _]
          tunnel: [w557 McPherson_Status.ctt."Scanning" ("McPherson Status")] -> w544
          tunnel: w536 -> [w556 w577]
          tunnel: [w555 w578] -> w545
          tunnel: w542 -> [_ w575]
          tunnel: [w552 w575] -> w541
          tunnel: w540 -> [w553 _]
          tunnel: w538 -> [w551 _]
          tunnel: w537 -> [w550 w573]
          frame False {
            # "+slew not done yet\nCheck pause"
            n184 = case shown="False" w558 {
              tunnel: [McPherson_Status.ctt."+Slew to Start" ("McPherson Status") McPherson_Status.ctt."Slew Pause" ("McPherson Status")] -> w557
              tunnel: w556 -> [w561 w567]
              tunnel: [w561 w566] -> w555
              tunnel: w554 -> [_ w565]
              tunnel: w553 -> [w560 _]
              tunnel: [w560 _] -> w552
              tunnel: w551 -> [w559 _]
              tunnel: w550 -> [_ w563]
              frame False {
                n185 = Wait Until Next ms Multiple(millisecond multiple=w559) -> ()  [unwired: 1 out]
              }
              frame True {
                n186 = call "McPherson Set X V.vi"("VISA Resource Name"=w565, "milliseconds to wait"=w563, "error In"=w567, "Action"=enum16{"Stop", "MoveTo", "SpeedAt"}."Stop") -> ("error out"=w566:errorcluster)  [unwired: 1 in, 2 out]
              }
            }
          }
          frame True {
            # "+slew done"
            n187 = local read "Begin"() -> (w570:dbl)
            n188 = local read "End"() -> (w569:dbl)
            n189 = Max & Min(x=w570, y=w569) -> (max(x,y)=w572:dbl, min(x,y)=w571:dbl)
            n190 = property on="Lambda Chart" class="WFChart (strict)"("Y Scale.Range:Maximum"=w572, "Y Scale.Range:Minimum"=w571) -> ()  [unwired: 2 in, 2 out]
            n191 = call "McPherson Set X V.vi"("VISA Resource Name"=w576, "milliseconds to wait"=w573, "SetValue In"=w575, "error In"=w577, "Action"=enum16{"Stop", "MoveTo", "SpeedAt"}."SpeedAt") -> ("error out"=w578:errorcluster)  [unwired: 2 out]
          }
        }
        n192 = Select(t=McPherson_Status.ctt."Cancel" ("McPherson Status"), s=w529, f=w544) -> (s? t:f=w533:T1)
      }
      frame "Scanning" {
        # "Scanning\nMay need timing"
        # "(Z0-Z2) * (Z1 -Z2) : >0 Scan Not done yet; <0 Scan done"
        n193 = Unbundle By Name(w595) -> ("BeginStep"=w594:i32, "EndStep"=w593:i32, "Speed Output"=w592:i16)
        n194 = Subtract(x=w586, y=w593) -> (x-y=w605:i32)
        n195 = Subtract(x=w594, y=w593) -> (x-y=w604:i32)
        n196 = To Double Precision Float(number=w605) -> (double precision float=w601:dbl)
        n197 = To Double Precision Float(number=w604) -> (double precision float=w600:dbl)
        n198 = Multiply(x=w601, y=w600) -> (x*y=w599:dbl)
        n199 = call "CheckCancel.vi"() -> ("Cancelled"=w583:bool)  [unwired: 2 in, 1 out]
        n200 = Greater Or Equal To 0?(x=w599) -> (x >= 0?=w598:bool)
        n201 = case shown="False" w598 {
          tunnel: w588 -> [w612 w620]
          tunnel: w587 -> [w611 w619]
          tunnel: [w610 w618] -> w606
          tunnel: w603 -> [_ w621]
          tunnel: [McPherson_Status.ctt."Scan Done" ("McPherson Status") w617] -> w596
          tunnel: w592 -> [_ w616]
          tunnel: [_ w615] -> w591
          tunnel: w590 -> [_ w614]
          tunnel: w589 -> [w607 w613]
          frame False {
            n202 = call "McPherson Set X V.vi"("VISA Resource Name"=w611, "milliseconds to wait"=w607, "error In"=w612, "Action"=enum16{"Stop", "MoveTo", "SpeedAt"}."Stop") -> ("error out"=w610:errorcluster)  [unwired: 1 in, 2 out]
          }
          frame True {
            # "Check Pause"
            n203 = case shown="False" w621 {
              tunnel: w620 -> [w625 w631]
              tunnel: w619 -> [_ w630]
              tunnel: [w625 w629] -> w618
              tunnel: [McPherson_Status.ctt."Scanning" ("McPherson Status") McPherson_Status.ctt."Scan Pause" ("McPherson Status")] -> w617
              tunnel: [w623 _] -> w615
              tunnel: w616 -> [w623 _]
              tunnel: w614 -> [w622 _]
              tunnel: w613 -> [_ w626]
              frame False {
                n204 = Wait Until Next ms Multiple(millisecond multiple=w622) -> ()  [unwired: 1 out]
              }
              frame True {
                # "Paused"
                n205 = call "McPherson Set X V.vi"("VISA Resource Name"=w630, "milliseconds to wait"=w626, "error In"=w631, "Action"=enum16{"Stop", "MoveTo", "SpeedAt"}."Stop") -> ("error out"=w629:errorcluster)  [unwired: 1 in, 2 out]
              }
            }
          }
        }
        n206 = Or(x=w582, y=w583) -> (x .or. y?=w581:bool)
        n207 = Select(t=McPherson_Status.ctt."Cancel" ("McPherson Status"), s=w581, f=w596) -> (s? t:f=w585:T1)
      }
      frame "Scan Done" {
        w643 = u8 0 ("Disabled")
        w634 = FALSE ("Visible")
        w633 = FALSE ("Visible")
        # "Update everything,\n\nIncluding the goto position"
        n208 = case shown="False" "Stop@End?" {
          selector: "Stop@End?" -> [_ w653]
          tunnel: [McPherson_Status.ctt."Standby" ("McPherson Status") McPherson_Status.ctt."Start Slew" ("t")] -> w646
          frame False {
            n209 = flat-sequence {
              frame #0 {
                n210 = Wait (ms)(milliseconds to wait=u32 100) -> ()  [unwired: 1 out]
              }
              frame #1 {
                w651 = u16 0 items=["Moving", "Calibration", "Key in", "Initialization"] ("Set Method")
                n211 = global read "gSpectrometer.vi" "Current Counter Position"() -> (w650:dbl)
                n212 = global read "gSpectrometer.vi" "CurrentStepperPosition"() -> (w649:i32)
                n213 = call "Load_McP_CounterPos.dat.VI"() -> ("Last Calibration Date"=w652:string)  [unwired: 1 in, 2 out]
                n214 = call "Save McP CounterPos.dat.VI"("Last Calibration Date"=w652, "Set Method"=w651, "McP Stepper Position"=w649, "McP Counter Position"=w650) -> ()  [unwired: 2 in, 1 out]
              }
            }
          }
          frame True {
            n215 = local write "PostScanSlew?"(w653) -> ()
          }
        }
        n216 = call "CheckCancel.vi"() -> ("Cancelled"=w638:bool)  [unwired: 2 in, 1 out]
        n217 = Or(x=w637, y=w638) -> (x .or. y?=w636:bool)
        n218 = property on="Scan" class="Bool"("Disabled"=w643) -> ()  [unwired: 2 in, 2 out]
        n219 = property on="Slew" class="Bool"("Disabled"=w643) -> ()  [unwired: 2 in, 2 out]
        n220 = property on="Pause" class="Bool (strict)"("Visible"=w633, "Value"=w633) -> ()  [unwired: 2 in, 2 out]
        n221 = Select(t=McPherson_Status.ctt."Cancel", s=w636, f=w646) -> (s? t:f=w640:T1)
        n222 = property on="Cancel" class="Bool (strict)"("Visible"=w634, "Value"=w634) -> ()  [unwired: 2 in, 2 out]
      }
      frame "Scan Pause" {
        n223 = case shown="False" w667 {
          tunnel: w671 -> [w680 w683]
          tunnel: w670 -> [w679 _]
          tunnel: [w678 w683] -> w669
          tunnel: [McPherson_Status.ctt."Update Z0" ("Prior Status") w681] -> w661
          tunnel: w664 -> [w676 _]
          tunnel: [w675 _] -> w663
          tunnel: w662 -> [w673 w682]
          tunnel: [McPherson_Status.ctt."Scanning" ("Prior Status") w681] -> w660
          frame False {
            n224 = Unbundle By Name(w676) -> ("Speed Output"=w675:i16)
            n225 = call "McPherson Set X V.vi"("VISA Resource Name"=w679, "milliseconds to wait"=w673, "SetValue In"=w675, "error In"=w680, "Action"=enum16{"Stop", "MoveTo", "SpeedAt"}."SpeedAt") -> ("error out"=w678:errorcluster)  [unwired: 2 out]
          }
          frame True {
            w681 = McPherson_Status.ctt."Scan Pause" ("Prior Status")
            n226 = Wait (ms)(milliseconds to wait=w682) -> ()  [unwired: 1 out]
          }
        }
        n227 = call "CheckCancel.vi"() -> ("Cancelled"=w658:bool)  [unwired: 2 in, 1 out]
        n228 = Or(x=w657, y=w658) -> (x .or. y?=w656:bool)
        n229 = Select(t=McPherson_Status.ctt."Cancel" ("McPherson Status"), s=w656, f=w661) -> (s? t:f=w666:T1)
      }
      frame "Slew Pause" {
        n230 = case shown="False" w697 {
          tunnel: w700 -> [w709 w712]
          tunnel: w699 -> [w708 _]
          tunnel: [w707 w712] -> w698
          tunnel: w693 -> [w706 _]
          tunnel: [McPherson_Status.ctt."Update Z0" ("Prior Status") w710] -> w694
          tunnel: w692 -> [w705 _]
          tunnel: [w705 _] -> w691
          tunnel: w690 -> [w703 w711]
          tunnel: [w702 w710] -> w689
          frame False {
            n231 = call "McPherson Set X V.vi"("VISA Resource Name"=w708, "milliseconds to wait"=w703, "SetValue In"=w706, "error In"=w709, "Action"=enum16{"Stop", "MoveTo", "SpeedAt"}."MoveTo") -> ("error out"=w707:errorcluster)  [unwired: 2 out]
            n232 = local read "Prior Status"() -> (w702:T1)
          }
          frame True {
            w710 = McPherson_Status.ctt."Slew Pause" ("Prior Status")
            n233 = Wait (ms)(milliseconds to wait=w711) -> ()  [unwired: 1 out]
          }
        }
        n234 = call "CheckCancel.vi"() -> ("Cancelled"=w687:bool)  [unwired: 2 in, 1 out]
        n235 = Or(x=w686, y=w687) -> (x .or. y?=w685:bool)
        n236 = Select(t=McPherson_Status.ctt."Cancel" ("McPherson Status"), s=w685, f=w694) -> (s? t:f=w696:T1)
      }
      frame "Cancel" {
        w720 = u8 0 ("Disabled")
        w714 = FALSE ("Visible")
        w713 = FALSE ("Visible")
        # "Use \"Slew Done\" only to save the position file!"
        n237 = call "McPherson Set X V.vi"("VISA Resource Name"=w724, "milliseconds to wait"=w721, "error In"=w725, "Action"=enum16{"Stop", "MoveTo", "SpeedAt"}."Stop") -> ("error out"=w718:errorcluster)  [unwired: 1 in, 2 out]
        n238 = property on="Slew" class="Bool"("Disabled"=w720) -> ()  [unwired: 2 in, 2 out]
        n239 = property on="Scan" class="Bool"("Disabled"=w720) -> ()  [unwired: 2 in, 2 out]
        n240 = property on="Pause" class="Bool (strict)"("Visible"=w713, "Value"=w713) -> ()  [unwired: 2 in, 2 out]
        n241 = property on="Cancel" class="Bool (strict)"("Visible"=w714, "Value"=w714) -> ()  [unwired: 2 in, 2 out]
      }
      frame "Update Z0" {
        n242 = local read "Scan Speed"() -> (w730:i32)
        n243 = flat-sequence {
          tunnel: w741 -> [w764]
          tunnel: w744 -> [w765]
          tunnel: w745 -> [w766]
          tunnel: [w766] -> w740
          tunnel: [w765] -> w739
          tunnel: [w764] -> w738
          tunnel: [w770] -> w743
          tunnel: [w767] -> w731
          tunnel: w740 -> [w772]
          tunnel: w739 -> [w771]
          tunnel: w738 -> [w769]
          frame #0 {
            n244 = Wait Until Next ms Multiple(millisecond multiple=u32 5) -> ()  [unwired: 1 out]
          }
          frame #1 {
            n245 = call "McPherson get status.vi"("Status"=T9."Position(Z0)", "error in (no error)"=w771, "Wait(ms)"=w769, "VISA Resource Name"=w772) -> ("error out"=w770:errorcluster, "CurrentPosition"=w767:i32)  [unwired: 1 in, 2 out]
          }
        }
        n246 = Not Equal?(x=w735, y=McPherson_Status.ctt."Update Z0") -> (x != y?=w736:bool)
        n247 = Select(t=w735, s=w736, f=McPherson_Status.ctt."Standby") -> (s? t:f=w726:T1)
        n248 = stacked-sequence {
          tunnel: w731 -> [w751 _]
          tunnel: w733 -> [_ w761]
          tunnel: [_ w760] -> w732
          tunnel: w730 -> [w755 _]
          tunnel: w729 -> [w754 _]
          tunnel: w728 -> [w753 _]
          tunnel: w727 -> [w752 _]
          tunnel: w726 -> [w747 _]
          frame #0 {
            n249 = local read "Grating  (g/mm)"() -> (w758:T3)
            n250 = local read "Wavelength Unit"() -> (w757:T4)
            n251 = call "McP_Step-WL_Converter.vi"("Wavelength Unit"=w757, "Option (Z0 <=> WL)"=enum16{"Z0 => WL", "WL => Z0", "Update WL only"}."Z0 => WL", "Grating Density"=w758, "Velocity (Steps/s)"=w755, "Stepper Position Input"=w751) -> ("Wavelength Output"=w748:dbl, "Current Couter Position"=w749:dbl, "nm Output"=w750:dbl, "Slew Rate"=→"Speed":dbl)  [unwired: 3 in, 4 out]
            "CurrentPosition" <- w748
            "Counter Reading" <- w749
            "Lambda Chart" <- w748
            n252 = Bundle By Name(cluster=w752, "McPherson Status"=w747, "Current WL"=w748, "Current Counter"=w749, "Current nm"=w750, "StepperPos"=w751) -> (w746:T2)
            n253 = Send Notification(notification=w746, notifier=w754, error in (no error)=w753) -> ()  [unwired: 2 out]
            n254 = local write "Spectrometer Pos"(w746) -> ()
          }
          frame #1 {
            n255 = Tick Count (ms)() -> (millisecond timer value=w760:u32)
            n256 = Subtract(x=w760, y=w761) -> (x-y=→"Time Lapse (msec)":u32)
          }
        }
      }
      frame "Sleep" {
        w773 = u8 2 ("Disabled")
        n257 = stacked-sequence {
          frame #0 {
            n258 = call "Sleep.vi"() -> ("Wokeup"=w781:bool)  [unwired: 3 in]
            n259 = local write "SleepTimer Reset"(w781) -> ()
            n260 = local write "SleepTimer Reset"(FALSE ("SleepTimer Reset")) -> ()
          }
          frame #1 {
            w782 = u8 0 ("Disabled")
            n261 = property on="Slew" class="Bool"("Disabled"=w782) -> ()  [unwired: 2 in, 2 out]
            n262 = property on="Scan" class="Bool"("Disabled"=w782) -> ()  [unwired: 2 in, 2 out]
          }
        }
        n263 = property on="Slew" class="Bool"("Disabled"=w773) -> ()  [unwired: 2 in, 2 out]
        n264 = property on="Scan" class="Bool"("Disabled"=w773) -> ()  [unwired: 2 in, 2 out]
      }
    }
    "error out" <- w49
    "Scan Speed" <- w66
    "McPherson Status" <- w43
    n265 = Unbundle By Name(w49) -> ("status"=w53:bool)
    n266 = Not Equal?(x=McPherson_Status.ctt."--Quit--", y=w55) -> (x != y?=w52:bool)
    n267 = And(x=w52, y=w53) -> (x .and. y?=w51:bool)
    n268 = Select(t=McPherson_Status.ctt."Error", s=w51, f=w55) -> (s? t:f=w70:T1)
    n269 = To Long Integer(number=w74) -> (32bit integer=w73:i32)
  }
